vi "Array mit Null auffuellen.vi"(10 "Array":dbl[](array[numeric]) format="%#_18f") -> (2 "Array 2":dbl[](array[numeric]) format="%#_18f")   [LabVIEW 2020, in "Linearisierung v2.lvlib"]
uses:
  Linearisierung v2.lvlib
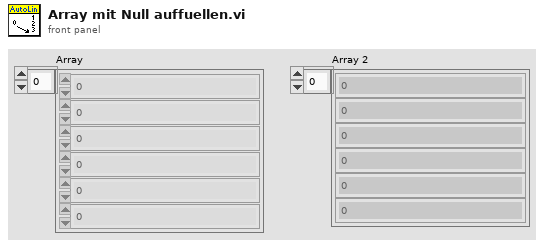
[diagram p1: front panel]
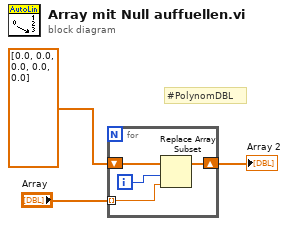
[diagram p0: block diagram]
diagram:
  # "#PolynomDBL"
  n1 = for {
    tunnel: "Array" -> [w6] mode=indexing
    shift-right: [w4] -> w1
    shift-left: sgl[] [0.0, 0.0, 0.0, 0.0, 0.0] -> [w7]
    i -> [w5]
    n2 = Replace Array Subset(array=w7, new element=w6, index=w5) -> (w4:sgl[])
  }
  "Array 2" <- w1
